vi "Create Element.vi"(8 "error in":errorcluster, 10 "Owner Document":refnum<k20>, 11 "Element in":refnum<class "Element.lvclass">) -> (0 "error out":errorcluster, 3 "Element out":refnum<class "Element.lvclass">)   [LabVIEW 2014, in "Element.lvclass"]
doc: "This vi is used to create an element with all the characteristics and properties that the element has. This vi should be used when saving a new xml document and the elements need to be created. The elements should be linked (parent child relationships given) after using this vi and before the xml document is saved."
uses:
  Element.lvclass
  <resource>/objmgr/DOMUserDefRef.rc
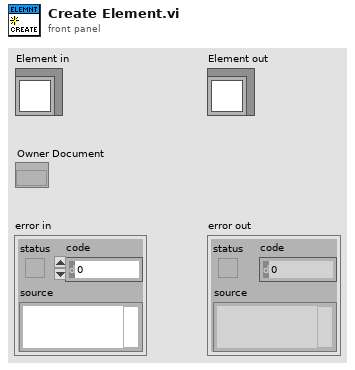
[diagram p1: front panel]
types:
  T1 = typedef "Attribute.ctl" = cluster{"Name":string, "Value":string}
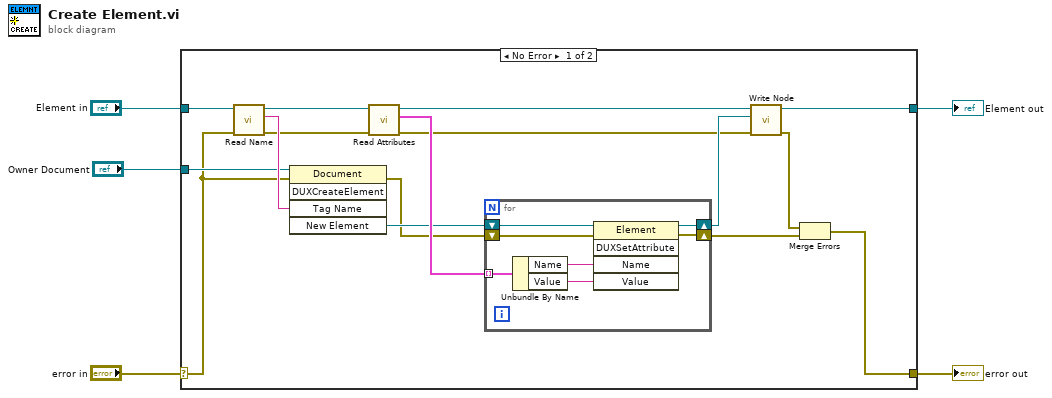
[diagram p0: block diagram]
diagram:
  n1 = case shown="No Error" "error in" {
    selector: "error in" -> [w7 w30]
    tunnel: [w6 w30] -> w4
    tunnel: [w12 w29] -> w2
    tunnel: "Element in" -> [w21 w29]
    tunnel: "Owner Document" -> [w13 _]
    frame No Error {
      n2 = call-dynamic "Read Name.vi"("error in"=w7, "Element in"=w21) -> ("error out"=w14:errorcluster, "Name"=w19:string, "Element out"=w20:refnum<class "Element.lvclass">)  [unwired: 7 in]
      n3 = invoke class="Document" method="DUXCreateElement"(reference=w13, error in=w7, "Tag Name"=w19) -> (error out=w15:errorcluster, "New Element"=w16:refnum<k20>)  [unwired: 2 in, 3 out]
      n4 = call-dynamic "Read Attributes.vi"("error in (no error)"=w14, "Element in"=w20) -> ("error out"=w10:errorcluster, "Attributes"=w17:T1[], "Element out"=w18:refnum<class "Element.lvclass">)  [unwired: 7 in]
      n5 = for {
        tunnel: w17 -> [w26] mode=indexing
        shift-right: [w27] -> w11
        shift-left: w16 -> [w28]
        shift-right: [w22] -> w8
        shift-left: w15 -> [w23]
        n6 = Unbundle By Name(w26) -> ("Name"=w25:string, "Value"=w24:string)
        n7 = invoke class="Element" method="DUXSetAttribute"(reference=w28, error in=w23, "Name"=w25, "Value"=w24) -> (reference out=w27:refnum<k20>, error out=w22:errorcluster)  [unwired: 1 in, 3 out]
      }
      n8 = call-dynamic "Write Node.vi"("error in"=w10, "Node"=w11, "Element in"=w18) -> ("error out"=w9:errorcluster, "Element out"=w12:refnum<class "Element.lvclass">)  [unwired: 7 in]
      n9 = Merge Errors(w9, w8) -> (w6:errorcluster)
    }
    frame Error {
    }
  }
  "error out" <- w4
  "Element out" <- w2
